vi "IMAQdx Sequence.vi"(8 "error in":errorcluster, 10 "Images In":T1[](array[typedef]), 11 "Session In":T2) -> (0 "error out":errorcluster, 2 "Images Out":T1[](array[typedef]), 3 "Session Out":T2)   [LabVIEW 2020, in "NI_Vision_Acquisition_Software.lvlib"]
doc: "Configures, starts, acquires, stops, and unconfigures a sequence acquisition. Use this VI to capture multiple images. If you call this VI before calling the IMAQdx Open Camera VI, the IMAQdx Sequence VI uses cam0 by default."
uses:
  NI_Vision_Acquisition_Software.lvlib
  IMAQdx.ctl
  IMAQ Image.ctl
  IMAQdx Acquisition Mode.ctl
  IMAQdx Buffer Number Mode.ctl
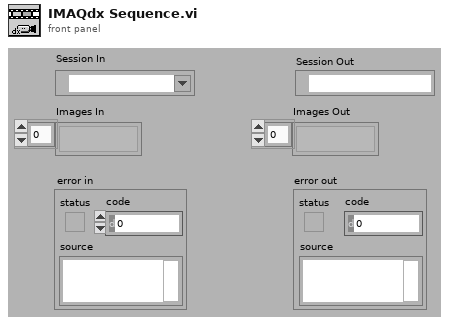
[diagram p1: front panel]
types:
  T1 = typedef "IMAQ Image.ctl" = refnum<image>
  T2 = typedef "IMAQdx.ctl" = refnum<k21>
  T3 = typedef "NI_Vision_Acquisition_Software.lvlib/IMAQdx Buffer Number Mode.ctl" = enum32{"Next", "Last", "Buffer Number", "Every", "Last New"}
  T4 = typedef "NI_Vision_Acquisition_Software.lvlib/IMAQdx Acquisition Mode.ctl" = enum32{"One Shot", "Continuous"}
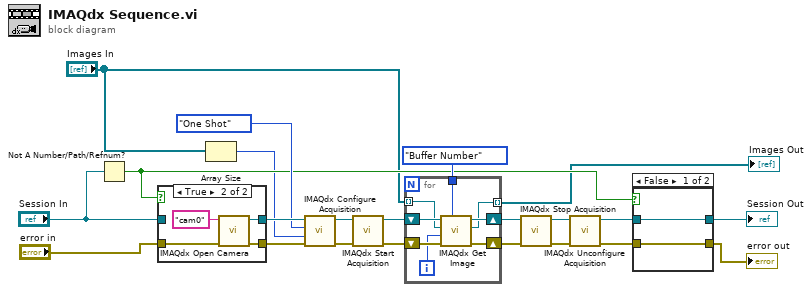
[diagram p0: block diagram]
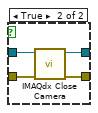
[diagram p2: hidden frame]
diagram:
  n1 = Not A Number/Path/Refnum?(number/path/refnum="Session In") -> (NaN/Path/Refnum?=w6:bool)
  n2 = case shown="True" w6 {
    tunnel: [w24 w28] -> w22
    tunnel: "Session In" -> [w24 _]
    tunnel: [w23 w27] -> w20
    tunnel: "error in" -> [w23 w26]
    frame False {
    }
    frame True {
      n3 = call "IMAQdx Open Camera.vi"("error in"=w26, "Session In"="cam0") -> ("error out"=w27:errorcluster, "Session Out"=w28:T2)  [unwired: 8 in]
    }
  }
  n4 = Array Size(array="Images In") -> (size(s)=w3:i32)
  n5 = call "IMAQdx Configure Acquisition.vi"("error in"=w20, "Number of Buffers"=w3, "Continuous?"=IMAQdx_Acquisition_Mode."One Shot", "Session In"=w22) -> ("error out"=w16:errorcluster, "Session Out"=w17:T2)  [unwired: 6 in]
  n6 = call "IMAQdx Start Acquisition.vi"("error in"=w16, "Session In"=w17) -> ("error out"=w14:errorcluster, "Session Out"=w15:T2)  [unwired: 8 in]
  n7 = for {
    tunnel: IMAQdx_Buffer_Number_Mode."Buffer Number" ("Buffer Number Mode") -> [w34]
    shift-right: [w32] -> w11
    shift-left: w14 -> [w35]
    shift-right: [w33] -> w12
    shift-left: w15 -> [w36]
    tunnel: "Images In" -> [w30] mode=indexing
    tunnel: [w29] -> w1 mode=indexing
    i -> [w31]
    n8 = call "IMAQdx Get Image.vi"("Buffer Number Mode (Next)"=w34, "error in"=w35, "Buffer Number In"=w31, "Image In"=w30, "Session In"=w36) -> ("error out"=w32:errorcluster, "Image Out"=w29:T1, "Session Out"=w33:T2)  [unwired: 3 in, 1 out]
  }
  "Images Out" <- w1
  n9 = call "IMAQdx Stop Acquisition.vi"("error in"=w11, "Session In"=w12) -> ("error out"=w9:errorcluster, "Session Out"=w10:T2)  [unwired: 8 in]
  n10 = call "IMAQdx Unconfigure Acquisition.vi"("error in"=w9, "Session In"=w10) -> ("error out"=w8:errorcluster, "Session Out"=w7:T2)  [unwired: 8 in]
  n11 = case shown="False" w6 {
    tunnel: w8 -> [w37 w41]
    tunnel: w7 -> [w38 w39]
    tunnel: [w38 w39] -> w5
    tunnel: [w37 w40] -> w4
    frame False {
    }
    frame True {
      n12 = call "IMAQdx Close Camera.vi"("error in"=w41, "Session In"=w39) -> ("error out"=w40:errorcluster)  [unwired: 9 in]
    }
  }
  "Session Out" <- w5
  "error out" <- w4
